vi "niFPGA I32xI32 MAC - MSB.vi"(5 "A":i32, 7 "B":i32, 9 "C":fxp<+/-,64,32>) -> (8 "A*B+C":i32=2838 format="%08x")   [LabVIEW 2017]
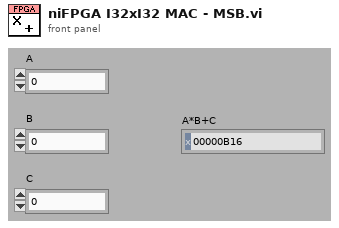
[diagram p1: front panel]
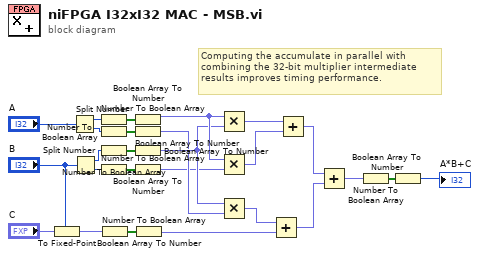
[diagram p0: block diagram]
diagram:
  # "Computing the accumulate in parallel with \ncombining the 32-bit multiplier intermediate \nresults improves timing performance."
  n1 = To Fixed-Point(fixed-point type="B", number="C") -> (fixed-point=w21:fxp<+/-,32,32>)
  n2 = Split Number(x="A") -> (hi(x)=w18:u16, lo(x)=w8:u16)
  n3 = Split Number(x="B") -> (hi(x)=w15:u16, lo(x)=w10:u16)
  n4 = Number To Boolean Array(number=w18) -> (Boolean array=w19:bool[])
  n5 = Number To Boolean Array(number=w8) -> (Boolean array=w13:bool[])
  n6 = Number To Boolean Array(number=w15) -> (Boolean array=w16:bool[])
  n7 = Number To Boolean Array(number=w10) -> (Boolean array=w11:bool[])
  n8 = Number To Boolean Array(number=w21) -> (Boolean array=w5:bool[])
  n9 = Boolean Array To Number(Boolean array=w19) -> (number=w17:fxp<+/-,16,0>)
  n10 = Boolean Array To Number(Boolean array=w13) -> (number=w12:fxp<+,16,-16>)
  n11 = Boolean Array To Number(Boolean array=w16) -> (number=w14:fxp<+/-,16,0>)
  n12 = Boolean Array To Number(Boolean array=w11) -> (number=w9:fxp<+,16,-16>)
  n13 = Boolean Array To Number(Boolean array=w5) -> (number=w4:fxp<+/-,32,0>)
  n14 = Multiply(x=w17, y=w14) -> (x*y=w26:fxp<+/-,32,0>)
  n15 = Multiply(x=w17, y=w9) -> (x*y=w7:fxp<+/-,16,-16>)
  n16 = Multiply(x=w14, y=w12) -> (x*y=w6:fxp<+/-,16,-16>)
  n17 = Add(x=w6, y=w4) -> (x+y=w22:fxp<+/-,33,1>)
  n18 = Add(x=w26, y=w7) -> (x+y=w25:fxp<+/-,32,0>)
  n19 = Add(x=w25, y=w22) -> (x+y=w2:fxp<+/-,32,0>)
  n20 = Number To Boolean Array(number=w2) -> (Boolean array=w3:bool[])
  n21 = Boolean Array To Number(Boolean array=w3) -> (number=→"A*B+C":i32)
